vi "libssh2_sftp_open_ex_r.vi"(5 "open_type (0 = file)":i32(ring) items=["File", "Directory"], 6 "attributes":T1, 7 "mode":i32(ring) items=["LIBSSH2_SFTP_S_IRWXU"=448, "LIBSSH2_SFTP_S_IRUSR"=256, "LIBSSH2_SFTP_S_IWUSR"=128, "LIBSSH2_SFTP_S_IXUSR"=64, "LIBSSH2_SFTP_S_IRWXG"=56, "LIBSSH2_SFTP_S_IRGRP"=32, "LIBSSH2_SFTP_S_IWGRP"=16, "LIBSSH2_SFTP_S_IXGRP"=8, "LIBSSH2_SFTP_S_IRWXO"=7, "LIBSSH2_SFTP_S_IROTH"=4, "LIBSSH2_SFTP_S_IWOTH"=2, "LIBSSH2_SFTP_S_IXOTH"=1], 8 "error in (no error)":errorcluster, 9 "flags":u32(ring) format="%x" items=["LIBSSH2_FXF_READ"=1, "LIBSSH2_FXF_WRITE"=2, "LIBSSH2_FXF_APPEND"=4, "LIBSSH2_FXF_CREAT"=8, "LIBSSH2_FXF_TRUNC"=16, "LIBSSH2_FXF_EXCL"=32], 10 "filename":string, 11 "sftp":T3) -> (0 "error out":errorcluster, 3 "sftp handle":T2)   [LabVIEW 2017, in "libssh2.lvlib"]
doc: "Open a file or directory handle for reading with custom flags and permissions."
uses:
  libssh2.lvlib
  SFTP Refnum.ctl
  SFTP Handle Refnum.ctl
  libssh2_sftp_attributes.ctl
  Acquire Session.vi
  Release Session.vi
  Not An SFTP Refnum.vi
  <vilib>/Utility/error.llb/Error Cluster From Error Code.vi
  Global Settings.vi
  Read SFTP Refnum.vi
  Read Session Refnum.vi
  <vilib>/Utility/semaphor.llb/Acquire Semaphore.vi
  <vilib>/Utility/semaphor.llb/Release Semaphore.vi
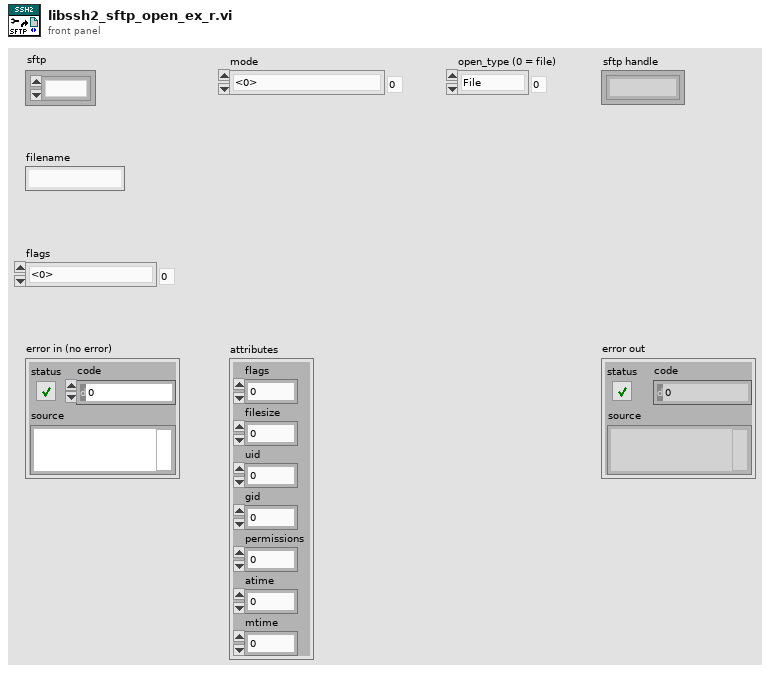
[diagram p1: front panel]
types:
  T1 = typedef "libssh2.lvlib/libssh2_sftp_attributes.ctl" = cluster{"flags":u32, "filesize":u64, "uid":u32, "gid":u32, "permissions":u32, "atime":u32, "mtime":u32}
  T2 = typedef "libssh2.lvlib/SFTP Handle Refnum.ctl" = refnum<k1>
  T3 = typedef "libssh2.lvlib/SFTP Refnum.ctl" = refnum<k1>
  T4 = cluster{"flags":u32, "<padding1>":u32, "filesize":u64, "uid":u32, "gid":u32, "permissions":u32, "atime":u32, "mtime":u32, "<padding2>":u32}
  T5 = cluster{"flags":u32, "<padding1>":u32, "filesize":u64, "uid":u32, "<padding2>":u32, "gid":u32, "<padding3>":u32, "permissions":u32, "<padding4>":u32, "atime":u32, "<padding5>":u32, "mtime":u32, "<padding6>":u32}
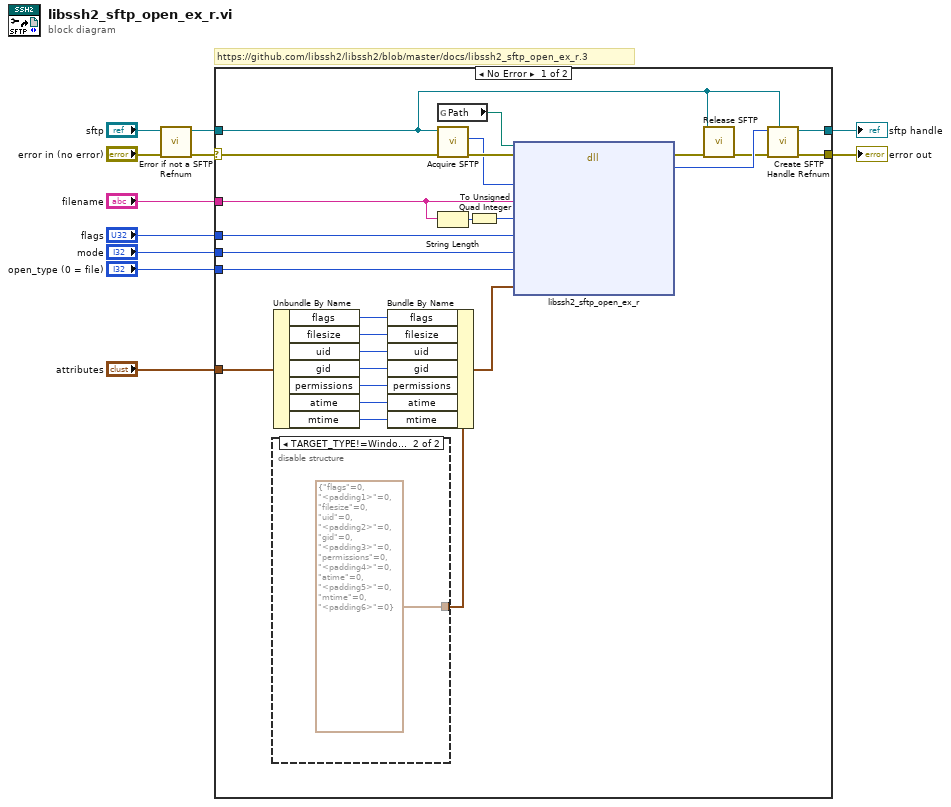
[diagram p0: block diagram]
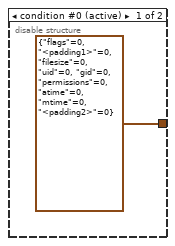
[diagram p2: hidden frame]
diagram:
  # "https://github.com/libssh2/libssh2/blob/master/docs/libssh2_sftp_open_ex_r.3"
  n1 = call "Error if not a SFTP Refnum.vi"("error in (no error)"="error in (no error)", "sftp"="sftp") -> ("error out"=w10:errorcluster, "sftp out"=w9:T3)  [unwired: 8 in]
  n2 = case shown="No Error" w10 {
    selector: w10 -> [w36 w40]
    tunnel: w9 -> [w13 _]
    tunnel: [w32 w40] -> w8
    tunnel: [w30 _] -> w2
    tunnel: "filename" -> [w29 _]
    tunnel: "flags" -> [w26 _]
    tunnel: "mode" -> [w25 _]
    tunnel: "open_type (0 = file)" -> [w24 _]
    tunnel: "attributes" -> [w23 _]
    frame No Error {
      n3 = disable-structure shown="TARGET_TYPE!=Windows&&TARGET_BITNESS==64" {
        disable-tunnel: [T4 {"flags"=0, "<padding1>"=0, "filesize"=0, "uid"=0, "gid"=0, "permissions"=0, "atime"=0, "mtime"=0, "<padding2>"=0} ("attrs") T5 {"flags"=0, "<padding1>"=0, "filesize"=0, "uid"=0, "<padding2>"=0, "gid"=0, "<padding3>"=0, "permissions"=0, "<padding4>"=0, "atime"=0, "<padding5>"=0, "mtime"=0, "<padding6>"=0} ("attrs")] -> w12
        frame condition #0 (active) {
        }
        frame condition #1 {
        }
      }
      n4 = Unbundle By Name(w23) -> ("flags"=w22:u32, "filesize"=w21:u64, "uid"=w19:u32, "gid"=w20:u32, "permissions"=w18:u32, "atime"=w17:u32, "mtime"=w16:u32)
      n5 = Bundle By Name(cluster=w12, "flags"=w22, "filesize"=w21, "uid"=w19, "gid"=w20, "permissions"=w18, "atime"=w17, "mtime"=w16) -> (w15:T4)
      n6 = global read "Global Settings.vi" "Path"() -> (w37:path)
      n7 = call "Acquire SFTP.vi"("error in (no error)"=w36, "sftp"=w13) -> ("error out"=w35:errorcluster, "LIBSSH2_SFTP*"=w34:u64)  [unwired: 8 in]
      n8 = String Length(string=w29) -> (length=w28:i32)
      n9 = To Unsigned Quad Integer(1:w28) -> (0:w27:u64)
      n10 = dll-call lib="?" fn="libssh2_sftp_open_ex_r"(path in=w37, error in=w35, "sftp"=w34, "filename"=w29, "filename_len"=w27, "flags"=w26, "mode"=w25, "open_type"=w24, "attrs"=w15) -> (error out=w33:errorcluster, "return value"=w31:u64)  [unwired: 8 in, 1 out]
      n11 = call "Release SFTP.vi"("error in (no error)"=w33, "sftp"=w13) -> ("error out"=w14:errorcluster)  [unwired: 9 in]
      n12 = call "Create SFTP Handle Refnum.vi"("sftp"=w13, "error in (no error)"=w14, "LIBSSH2_SFTP_HANDLE*"=w31) -> ("error out"=w32:errorcluster, "sftp handle"=w30:T2)  [unwired: 7 in]
    }
    frame Error {
    }
  }
  "error out" <- w8
  "sftp handle" <- w2
